vi "DevInit.vi"(4 "Ïµ½y î‘B":refnum<vi>, 6 "運行信息":refnum<vi>, 8 "错误输入（无错误）":errorcluster, 10 "所有的":cluster{"Addr":u8, "Enable?":bool}[](array[cluster]), 11 "DevControl输入":refnum<class "DevControl.lvclass">) -> (0 "error out":errorcluster)   [LabVIEW 2012]
uses:
  Fun/Dev/DevControl.lvclass
  SystemState.ctl
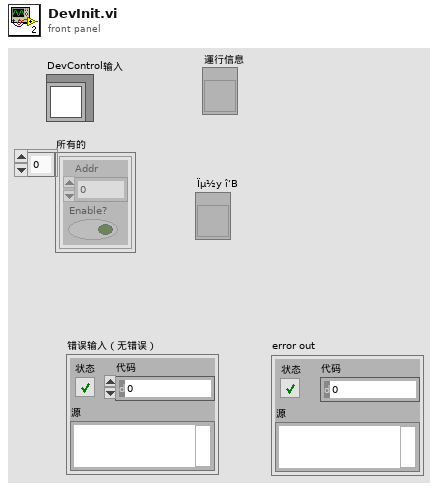
[diagram p1: front panel]
types:
  T1 = typedef "SystemState.ctl" = enum16{"Quit", "Error", "Stopping", "Starting", "Init", "Scan", "Menu", "ReadConf", "Idle"}
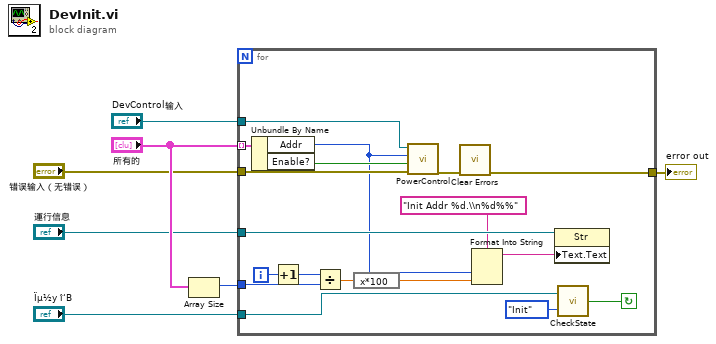
[diagram p0: block diagram]
diagram:
  n1 = Array Size(array="所有的") -> (size(s)=w6:i32)
  n2 = for {
    tunnel: "所有的" -> [w25] mode=indexing
    tunnel: "错误输入（无错误）" -> [w24]
    tunnel: "DevControl输入" -> [w23]
    tunnel: "運行信息" -> [w20]
    tunnel: w6 -> [w15]
    tunnel: "Ïµ½y î‘B" -> [w10]
    tunnel: [w8] -> w1
    i -> [w16]
    stop <- w11 continue-if-true
    n3 = Unbundle By Name(w25) -> ("Addr"=w18:u8, "Enable?"=w22:bool)
    n4 = Increment(x=w16) -> (x+1=w14:i32)
    n5 = Divide(x=w14, y=w15) -> (x/y=w13:dbl)
    n6 = expression code="x*100"(w13) -> (w12:dbl)
    n7 = call-dynamic "PowerControl.vi"("error in (no error)"=w24, "On/Off?"=w22, "Addr"=w18, "DevControl 输入"=w23) -> ("error out"=w21:errorcluster)  [unwired: 6 in, 1 out]
    n8 = call <vilib>:"Clear Errors.vi"("error in (no error)"=w21) -> ("error out"=w8:errorcluster)  [unwired: 6 in]
    n9 = Format Into String(format string="Init Addr %d.\\n%d%%" ("格式字符串"), w18, w12) -> (resulting string=w19:string)  [unwired: 2 in, 1 out]
    n10 = property class="Str"(reference=w20, "Text.Text"=w19) -> ()  [unwired: 1 in, 2 out]
    n11 = call "CheckState.vi"("™z²é î‘B"=SystemState."Init", "Ïµ½y î‘B"=w10) -> ("ChkOK?"=w11:bool)
  }
  "error out" <- w1
